vi "opt_pump_lineset_wait.vi"(8 "error in":errorcluster, 10 "True: Optically Pump False: Do nothing":bool, 11 "milliseconds to pump":u32=200) -> (0 "error out":errorcluster)   [LabVIEW 2012]
panel:
  in  "455 Pumping Time":u32=500
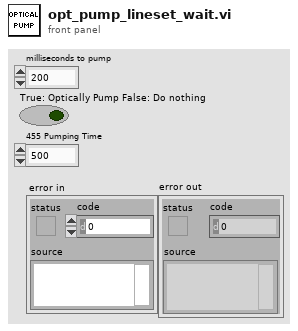
[diagram p1: front panel]
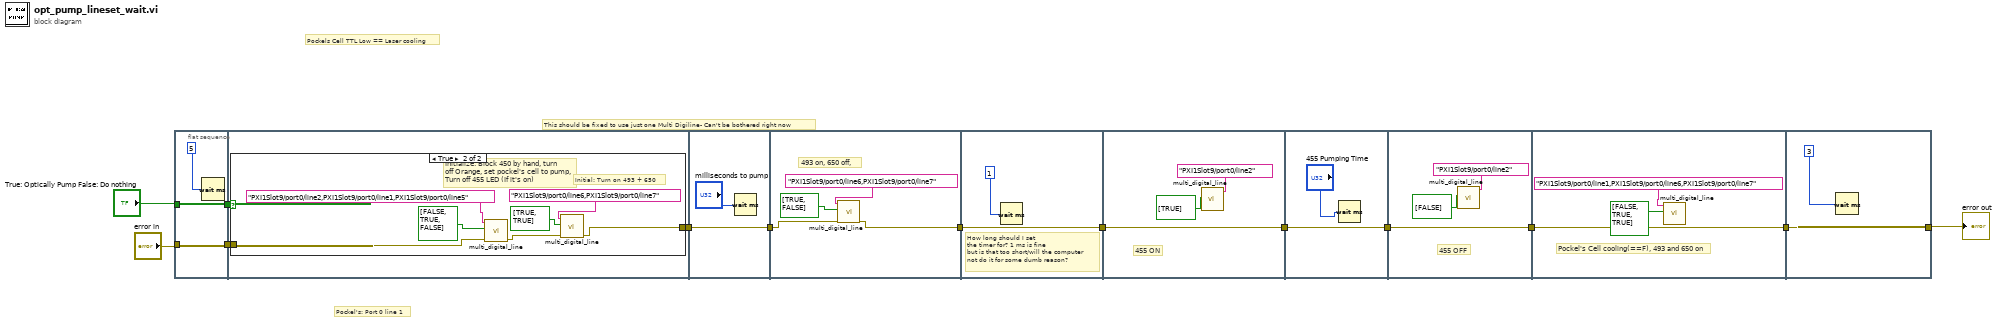
[diagram p0: block diagram]
diagram:
  # "Pockel's: Port 0 line 1"
  # "Pockels Cell TTL Low == Laser cooling"
  # "This should be fixed to use just one Multi Digiline- Can't be bothered right now"
  n1 = flat-sequence {
    tunnel: "True: Optically Pump False: Do nothing" -> [w15]
    tunnel: "error in" -> [w16]
    tunnel: [w16] -> w3
    tunnel: [w15] -> w2
    tunnel: [w18] -> w11
    tunnel: w3 -> [w19]
    tunnel: w2 -> [w17]
    tunnel: w11 -> [w29]
    tunnel: [w29] -> w9
    tunnel: w9 -> [w31]
    tunnel: [w30] -> w8
    tunnel: w8 -> [w35]
    tunnel: [w35] -> w7
    tunnel: w7 -> [w38]
    tunnel: [w38] -> w6
    tunnel: w6 -> [w40]
    tunnel: [w40] -> w5
    tunnel: w5 -> [w43]
    tunnel: [w43] -> w4
    tunnel: w4 -> [w46]
    tunnel: [w46] -> w1
    tunnel: [w48] -> w12
    tunnel: w1 -> [w48]
    frame #0 {
      n2 = Wait (ms)(milliseconds to wait=u32 5 ("milliseconds to pump 2")) -> ()  [unwired: 1 out]
    }
    frame #1 {
      n3 = case shown="True" w17 {
        tunnel: w19 -> [w20 w27]
        tunnel: [w20 w25] -> w18
        frame False {
        }
        frame True {
          # "Initial: Turn on 493 + 650"
          # "Initialize: Block 450 by hand, turn\noff Orange, set pockel's cell to pump,\nTurn off 455 LED (If it's on)"
          n4 = call "multi_digital_line.vi"("error in"=w27, "data"=bool[] [FALSE, TRUE, FALSE], "lines"=tag "PXI1Slot9/port0/line2,PXI1Slot9/port0/line1,PXI1Slot9/port0/line5" ("lines 2")) -> ("error out"=w26:errorcluster)  [unwired: 8 in]
          n5 = call "multi_digital_line.vi"("error in"=w26, "data"=bool[] [TRUE, TRUE], "lines"=tag "PXI1Slot9/port0/line6,PXI1Slot9/port0/line7" ("lines 2")) -> ("error out"=w25:errorcluster)  [unwired: 8 in]
        }
      }
    }
    frame #2 {
      n6 = Wait (ms)(milliseconds to wait="milliseconds to pump") -> ()  [unwired: 1 out]
    }
    frame #3 {
      # "493 on, 650 off,"
      n7 = call "multi_digital_line.vi"("error in"=w31, "data"=bool[] [TRUE, FALSE], "lines"=tag "PXI1Slot9/port0/line6,PXI1Slot9/port0/line7" ("lines 2")) -> ("error out"=w30:errorcluster)  [unwired: 8 in]
    }
    frame #4 {
      # "How long should I set\nthe timer for? 1 ms is fine\nbut is that too short/will the computer\nnot do it for some dumb reason?"
      n8 = Wait (ms)(milliseconds to wait=u32 1 ("milliseconds to pump 2")) -> ()  [unwired: 1 out]
    }
    frame #5 {
      # "455 ON"
      n9 = call "multi_digital_line.vi"("data"=bool[] [TRUE], "lines"=tag "PXI1Slot9/port0/line2" ("lines 2")) -> ()  [unwired: 9 in, 1 out]
    }
    frame #6 {
      n10 = Wait (ms)(milliseconds to wait="455 Pumping Time") -> ()  [unwired: 1 out]
    }
    frame #7 {
      # "455 OFF"
      n11 = call "multi_digital_line.vi"("data"=bool[] [FALSE], "lines"=tag "PXI1Slot9/port0/line2" ("lines 2")) -> ()  [unwired: 9 in, 1 out]
    }
    frame #8 {
      # "Pockel's Cell cooling(==F), 493 and 650 on"
      n12 = call "multi_digital_line.vi"("data"=bool[] [FALSE, TRUE, TRUE], "lines"=tag "PXI1Slot9/port0/line1,PXI1Slot9/port0/line6,PXI1Slot9/port0/line7" ("lines 2")) -> ()  [unwired: 9 in, 1 out]
    }
    frame #9 {
      n13 = Wait (ms)(milliseconds to wait=u32 3 ("455 Pumping Time 2")) -> ()  [unwired: 1 out]
    }
  }
  "error out" <- w12
